vi "Handle Userinfo.vi"(8 "error in (no error)":errorcluster, 10 "Name":string, 11 "LV Chat Client in":refnum<class "LV Chat Client.lvclass">) -> (0 "error out":errorcluster, 1 "Cancelled?":bool, 2 "Name Accepted?":bool, 3 "LV Chat Client out":refnum<class "LV Chat Client.lvclass">)   [LabVIEW 2020, in "LV Chat Client.lvclass"]
uses:
  LV Chat Client.lvclass
  LV Chat Client.lvclass/LV Chat Client.ctl
  <vilib>/event_ctls.llb/eventvkey.ctl
panel:
  out "Prompt":string
  in  "Cancel":bool
  in  "OK":bool
  in  "Name Input":string
  # "Clicking cancel will close the application."
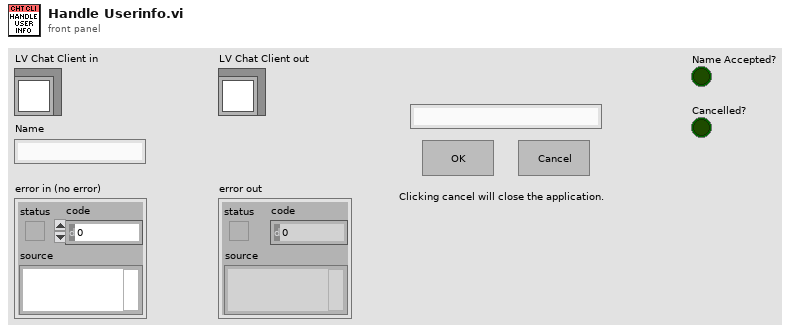
[diagram p1: front panel]
types:
  T1 = enum32{"Invalid", "Standard", "Closed", "Hidden", "Minimized", "Maximized"}
  T2 = typedef "eventvkey.ctl" = enum16{"ASCII", "Enter", "Return", "Shift", "Ctrl", "Alt", "Cmd", "Opt", "Caps", "NumLock", "Clear", "Break", "Up", "Down", "Left", "Right", "Insert", "Delete", "Home", "End", "PageUp", "PageDown", "Escape", "Help", "Pause", "ScrollLock", "F1", "F2", "F3", "F4", "F5", "F6", "F7", "F8", "F9", "F10", "F11", "F12", "F13", "F14", "F15", "F16", "F17", "F18", "F19", "F20", "F21", "F22", "F23", "F24", "Play", "VolumeUp", "VolumeDown", "Mute", "Two Byte Char"}
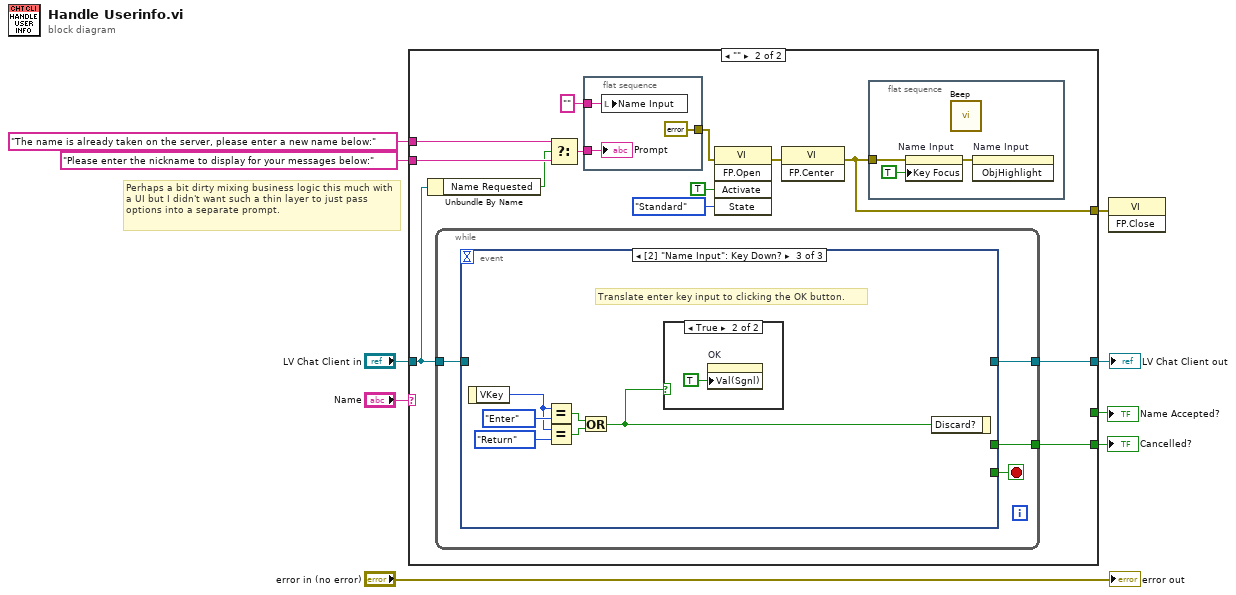
[diagram p0: block diagram]
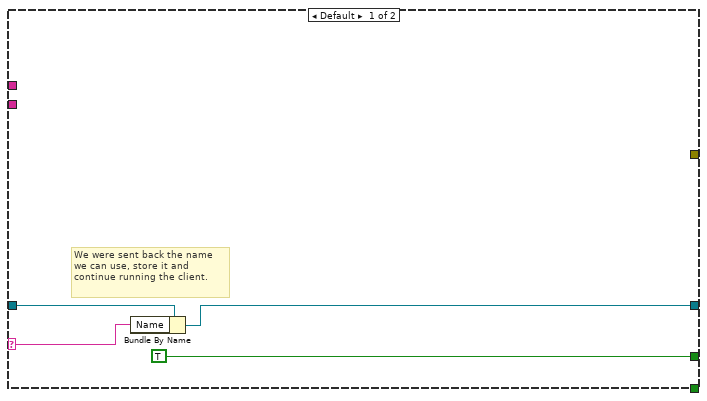
[diagram p2: hidden frame]
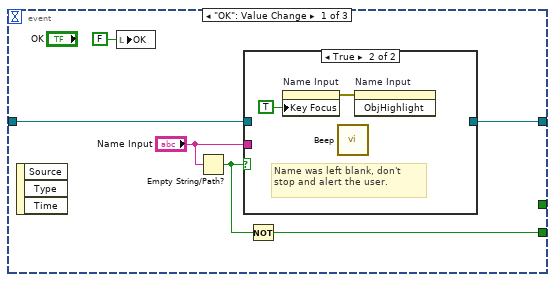
[diagram p3: hidden frame]
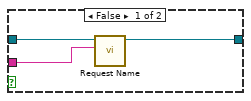
[diagram p4: hidden frame]
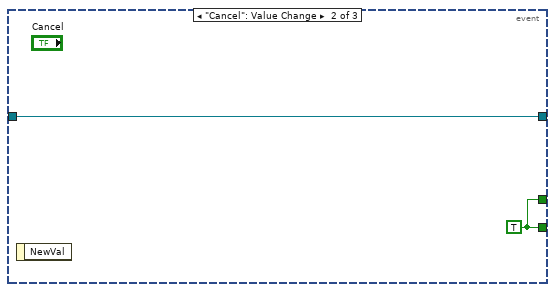
[diagram p5: hidden frame]
diagram:
  # "Perhaps a bit dirty mixing business logic this much with a UI but I didn't want such a thin layer to just pass options into a separate prompt."
  n1 = case shown="\"\"" "Name" {
    selector: "Name" -> [w12 _]
    tunnel: "LV Chat Client in" -> [w13 w18]
    tunnel: "The name is already taken on the server, please enter a new name below:" -> [_ w26]
    tunnel: "Please enter the nickname to display for your messages below:" -> [_ w25]
    tunnel: [_ w17] -> w4
    tunnel: [w11 w16] -> w3
    tunnel: [TRUE _] -> w2
    tunnel: [_ w14] -> w1
    frame Default {
      # "We were sent back the name we can use, store it and continue running the client."
      n2 = Bundle By Name(cluster=w13, "Name"=w12) -> (w11:refnum<class "LV Chat Client.lvclass">)
    }
    frame "" {
      n3 = Unbundle By Name(w18) -> ("Name Requested"=w24:bool)
      n4 = while {
        tunnel: w18 -> [w36]
        tunnel: [w34] -> w17
        tunnel: [w33] -> w16
        stop <- w35 stop-if-true
        n5 = event shown="[2] \"Name Input\": Key Down?" {
          selector: _ -> [_ _ _]
          dyn-events: _ -> [_ _ _]
          timeout: _ -> [_ _ _]
          tunnel: w36 -> [w39 w48 _]
          tunnel: [w42 w49 _] -> w35
          tunnel: [_ w49 _] -> w34
          tunnel: [w38 w48 _] -> w33
          event "OK": Value Change {
            n6 = event-data() -> ()  [unwired: 1 in, 3 out]
            n7 = local write "OK"(FALSE ("OK")) -> ()
            n8 = Empty String/Path?(string/path="Name Input") -> (empty?=w41:bool)
            n9 = case shown="True" w41 {
              tunnel: "Name Input" -> [w44 _]
              tunnel: w39 -> [w45 _]
              tunnel: [w43 _] -> w38
              frame False {
                n10 = call "Request Name.vi"("Name"=w44, "LV Chat Client in"=w45) -> ("LV Chat Client out"=w43:refnum<class "LV Chat Client.lvclass">)  [unwired: 8 in, 1 out]
              }
              frame True {
                # "Name was left blank, don't stop and alert the user."
                n11 = property on="Name Input" class="Str"("Key Focus"=TRUE) -> (error out=w46:errorcluster)  [unwired: 2 in, 1 out]
                n12 = call <vilib>:"Beep.vi"() -> ()  [unwired: 12 in]
                n13 = invoke on="Name Input" class="Str" method="ObjHighlight"(error in=w46) -> ()  [unwired: 2 in, 3 out]
              }
            }
            n14 = Not(x=w41) -> (.not. x?=w42:bool)
          }
          event "Cancel": Value Change {
            w49 = TRUE
            n15 = event-data() -> ()  [unwired: 1 in, 1 out]
          }
          event "Name Input": Key Down? {
            # "Translate enter key input to clicking the OK button."
            n16 = event-data() -> ("VKey"=w53:T2)  [unwired: 1 in]
            n17 = Equal?(x=w53, y=eventvkey."Enter" ("VKey")) -> (x = y?=w52:bool)
            n18 = Equal?(x=w53, y=eventvkey."Return" ("VKey")) -> (x = y?=w51:bool)
            n19 = Or(x=w52, y=w51) -> (x .or. y?=w50:bool)
            n20 = case shown="True" w50 {
              frame False {
              }
              frame True {
                n21 = property on="OK" class="Bool (strict)"("Val(Sgnl)"=TRUE ("Value (Signaling)")) -> ()  [unwired: 2 in, 2 out]
              }
            }
            n22 = event-data("Discard?"=w50) -> ()  [unwired: 1 in, 1 out]
          }
        }
      }
      n23 = Select(t=w26, s=w24, f=w25) -> (s? t:f=w23:string)
      n24 = flat-sequence {
        tunnel: w23 -> [w32]
        tunnel: [errorcluster {"status"=FALSE, "code"=0, "source"=""} ("error constant")] -> w19
        tunnel: "" -> [w30]
        frame #0 {
          n25 = local write "Name Input"(w30) -> ()
          "Prompt" <- w32
        }
      }
      n26 = invoke class="VI" method="FP.Open"(error in=w19, "Activate"=TRUE ("Activate?"), "State"=T1."Standard") -> (error out=w20:errorcluster)  [unwired: 2 in, 4 out]
      n27 = invoke class="VI" method="FP.Center"(error in=w20) -> (error out=w14:errorcluster)  [unwired: 2 in, 2 out]
      n28 = flat-sequence {
        tunnel: w14 -> [w29]
        frame #0 {
          n29 = property on="Name Input" class="Str"(error in=w29, "Key Focus"=TRUE) -> (error out=w27:errorcluster)  [unwired: 1 in, 1 out]
          n30 = call <vilib>:"Beep.vi"() -> ()  [unwired: 12 in]
          n31 = invoke on="Name Input" class="Str" method="ObjHighlight"(error in=w27) -> ()  [unwired: 2 in, 3 out]
        }
      }
    }
  }
  "LV Chat Client out" <- w3
  "Cancelled?" <- w4
  "Name Accepted?" <- w2
  n32 = invoke class="VI" method="FP.Close"(error in=w1) -> ()  [unwired: 2 in, 3 out]
  "error out" <- "error in (no error)"
